vi "CSVCreate.vi"(7 "Header":string, 8 "error in":errorcluster, 9 "Append File":refnum<vi>, 10 "Data Input":string, 11 "file path (dialog if empty)":path) -> (0 "error out":errorcluster, 3 "path 5":path)   [LabVIEW 2015]
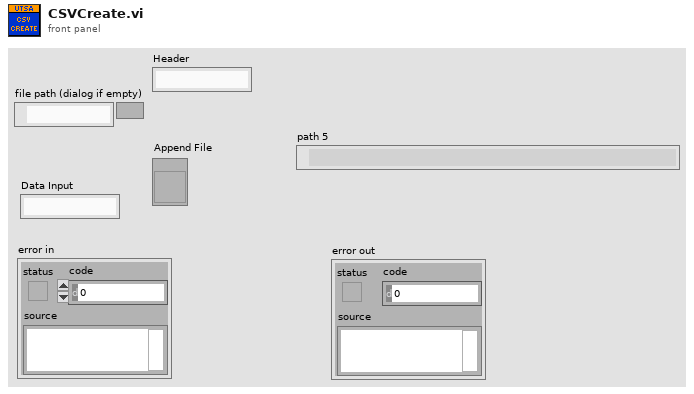
[diagram p1: front panel]
types:
  T1 = enum16{"open", "replace", "create", "open or create", "replace or create", "replace or create with confirmation"}
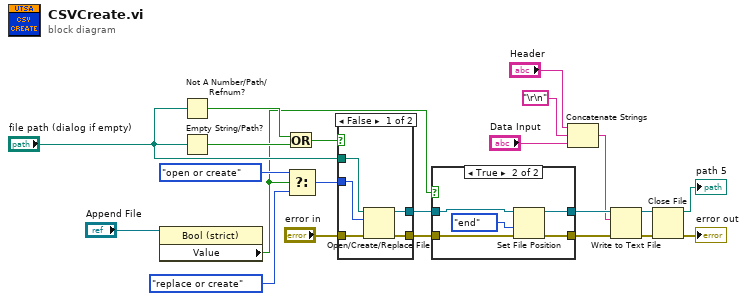
[diagram p0: block diagram]
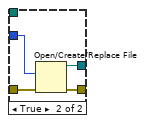
[diagram p3: hidden frame]
diagram:
  n1 = property class="Bool (strict)"(reference="Append File") -> ("Value"=w1:bool)  [unwired: 1 in, 2 out]
  n2 = Not A Number/Path/Refnum?(number/path/refnum="file path (dialog if empty)") -> (NaN/Path/Refnum?=w15:bool)
  n3 = Empty String/Path?(string/path="file path (dialog if empty)") -> (empty?=w16:bool)
  n4 = Or(x=w15, y=w16) -> (x .or. y?=w14:bool)
  n5 = Select ("function")(t=T1."open or create" ("operation (0:open)"), s=w1, f=T1."replace or create" ("operation (0:open)")) -> (s? t:f=w11:T1)
  n6 = case shown="False" w14 {
    tunnel: "error in" -> [w27 w30]
    tunnel: [w26 w31] -> w9
    tunnel: [w25 w29] -> w8
    tunnel: "file path (dialog if empty)" -> [w24 _]
    tunnel: w11 -> [w23 w28]
    frame False {
      n7 = Open/Create/Replace File(file path (use dialog)=w24, error in=w27, operation (0:open)=w23) -> (refnum out=w25:refnum<file>, error out=w26:errorcluster)  [unwired: 3 in, 1 out]
    }
    frame True {
      n8 = Open/Create/Replace File(error in=w30, operation (0:open)=w28) -> (refnum out=w29:refnum<file>, error out=w31:errorcluster)  [unwired: 4 in, 1 out]
    }
  }
  n9 = case shown="True" w1 {
    tunnel: w9 -> [w32 w38]
    tunnel: [w32 w37] -> w10
    tunnel: w8 -> [w33 w35]
    tunnel: [w33 w36] -> w7
    frame False {
    }
    frame True {
      n10 = Set File Position(refnum=w35, from (0:start)=enum16{"start", "end", "current"}."end", error in=w38) -> (refnum out=w36:refnum<file>, error out=w37:errorcluster)  [unwired: 1 in]
    }
  }
  n11 = Concatenate Strings("Header", "\r\n", "Data Input") -> (w3:string)
  n12 = Write to Text File(file (use dialog)=w7, text=w3, error in=w10) -> (refnum out=w18:refnum<file>, error out=w17:errorcluster)  [unwired: 1 in, 1 out]
  n13 = Close File(refnum=w18, error in=w17) -> (path=→"path 5":path, error out=→"error out":errorcluster)
